vi "cpu.vi"() -> (3 "load":dbl)   [LabVIEW 2019]
uses:
  <vilib>/NI_Real-Time Target Support.lvlib
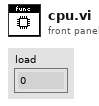
[diagram p1: front panel]
types:
  T1 = typedef "NI_Real-Time Target Support.lvlib/RT CPU Load.ctl" = cluster{"Total (%)":dbl, "Time Critical (%)":dbl, "Timed Structures (%)":dbl, "High (%)":dbl, "Above Normal (%)":dbl, "Normal (%)":dbl, "Background (%)":dbl, "Idle (%)":dbl, "ISR (%)":dbl}
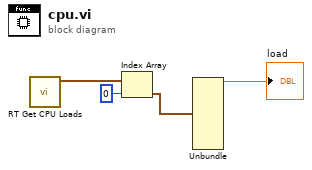
[diagram p0: block diagram]
diagram:
  n1 = call <vilib>:"RT Get CPU Loads.vi"() -> ("CPU loads"=w2:T1[])  [unwired: 10 in, 1 out]
  n2 = Index Array(array=w2, index=0) -> (element=w3:T1)
  n3 = Unbundle(w3) -> ("Total (%)"=→"load":dbl)  [unwired: 8 out]
